vi "STA - Wave V6 Host_Wait.vi"() -> ()   [LabVIEW 2015]
doc: "The continuous acquisition mode tells the FPGA to acquire points indefinitely until a stop command is issued or until an error is encountered (FIFO overflow, module underflow, and so on). \n\nIn this acquisition mode, explicitly call the appropriate rwfm_ConfigTiming VI and set the host application's data buffer to be many times larger than the read size. The examples use a 10X size by default. If the host application's data buffer fills, then the FPGA experiences a FIFO overflow causing the acquisition to stop."
uses:
  <vilib>/rvi/interface/nirviCloseFPGA/nirviCloseFPGA.xnode
  <vilib>/FPGAPlugInAG/Dynamic/niLvFpga_Close_Dynamic.vi
  <vilib>/NI/cRIO Wfm/cRIO Wfm.lvlib
  <vilib>/rvi/interface/nirviMethod/nirviMethod.xnode
  <vilib>/rvi/interface/nirviMethod/StockFPGA_InlinedMethodWaitForSingleIRQ.vi
  <vilib>/FPGAPlugInAG/Dynamic/niLvFpga_WaitOnIrq_Dynamic.vi
  <vilib>/rvi/interface/nirviOpenFPGA/nirviOpenFPGA.xnode
  C:/Program Files (x86)/National Instruments/LabVIEW 2015/ProjectTemplates/Source/cRIOWfm/FPGA/[FPGA] SAR Acq Main.vi
  D/Documents/LabVIEW Data/STA - Waveform V0/FPGA Bitfiles/SARAcqMain_9074.lvbitx
  FPGA Bitfiles/STA-WaveformV6_FPGATarget2_[FPGA]DeltaSigMa_RDSJJgoi1gU.lvbitx
  FPGA/[FPGA] DeltaSig Main V6_bis.vi
  <vilib>/FPGAPlugInAG/cRIO-9112/niLvFpga_Open_cRIO-9112.vi
  <vilib>/rvi/interface/common/dynamic/niFpgaDynamicAddResources.vi
panel:
  out "Channel Config":T1(array[cluster])=[{"Channel Name"="Mod1/a0", "Sensitivity mV_EU"=1000.0, "EU"="V", "dB Ref EU"=1.0}, {"Channel Name"="Mod1/a1", "Sensitivity mV_EU"=1000.0, "EU"="V", "dB Ref EU"=1.0}, {"Channel Name"="Mod1/a2", "Sensitivity mV_EU"=1000.0, "EU"="V", "dB Ref EU"=1.0}, {"Channel Name"="Mod1/a3", "Sensitivity mV_EU"=1000.0, "EU"="V", "dB Ref EU"=1.0}, {"Channel Name"="Mod2/a0", "Sensitivity mV_EU"=1000.0, "EU"="V", "dB Ref EU"=1.0}, {"Channel Name"="Mod2/a1", "Sensitivity mV_EU"=1000.0, "EU"="V", "dB Ref EU"=1.0}, {"Channel Name"="Mod2/a2", "Sensitivity mV_EU"=1000.0, "EU"="V", "dB Ref EU"=1.0}, {"Channel Name"="Mod2/a3", "Sensitivity mV_EU"=1000.0, "EU"="V", "dB Ref EU"=1.0}, {"Channel Name"="Mod3/a0", "Sensitivity mV_EU"=1000.0, "EU"="V", "dB Ref EU"=1.0}, {"Channel Name"="Mod3/a1", "Sensitivity mV_EU"=1000.0, "EU"="V", "dB Ref EU"=1.0}, {"Channel Name"="Mod3/a2", "Sensitivity mV_EU"=1000.0, "EU"="V", "dB Ref EU"=1.0}, {"Channel Name"="Mod3/a3", "Sensitivity mV_EU"=1000.0, "EU"="V", "dB Ref EU"=1.0}, {"Channel Name"="Mod4/a0", "Sensitivity mV_EU"=1000.0, "EU"="V", "dB Ref EU"=1.0}, {"Channel Name"="Mod4/a1", "Sensitivity mV_EU"=1000.0, "EU"="V", "dB Ref EU"=1.0}, {"Channel Name"="Mod4/a2", "Sensitivity mV_EU"=1000.0, "EU"="V", "dB Ref EU"=1.0}, {"Channel Name"="Mod4/a3", "Sensitivity mV_EU"=1000.0, "EU"="V", "dB Ref EU"=1.0}, {"Channel Name"="Mod5/a0", "Sensitivity mV_EU"=1000.0, "EU"="V", "dB Ref EU"=1.0}, {"Channel Name"="Mod5/a1", "Sensitivity mV_EU"=1000.0, "EU"="V", "dB Ref EU"=1.0}, {"Channel Name"="Mod5/a2", "Sensitivity mV_EU"=1000.0, "EU"="V", "dB Ref EU"=1.0}, {"Channel Name"="Mod5/a3", "Sensitivity mV_EU"=1000.0, "EU"="V", "dB Ref EU"=1.0}, {"Channel Name"="Mod6/a0", "Sensitivity mV_EU"=1000.0, "EU"="V", "dB Ref EU"=1.0}, {"Channel Name"="Mod6/a1", "Sensitivity mV_EU"=1000.0, "EU"="V", "dB Ref EU"=1.0}, {"Channel Name"="Mod6/a2", "Sensitivity mV_EU"=1000.0, "EU"="V", "dB Ref EU"=1.0}, {"Channel Name"="Mod6/a3", "Sensitivity mV_EU"=1000.0, "EU"="V", "dB Ref EU"=1.0}] caption="Channel Name      Scale [mV/EU]              EU                           dB Ref [EU]"
  out "Time Measure":dbl
  out "data rate (S/s)":u32
  out "Samples per Read":i32
  out "file path":path
  out "error out":errorcluster
  in  "stop":bool
  out "Waveform Graph":waveform(sgl)[](graph)
  out "Buffer Backlog":dbl caption="RT Buffer Backlog [%]" format="%#.2g"
  # "Sampling Info"
  # "Channel Info"
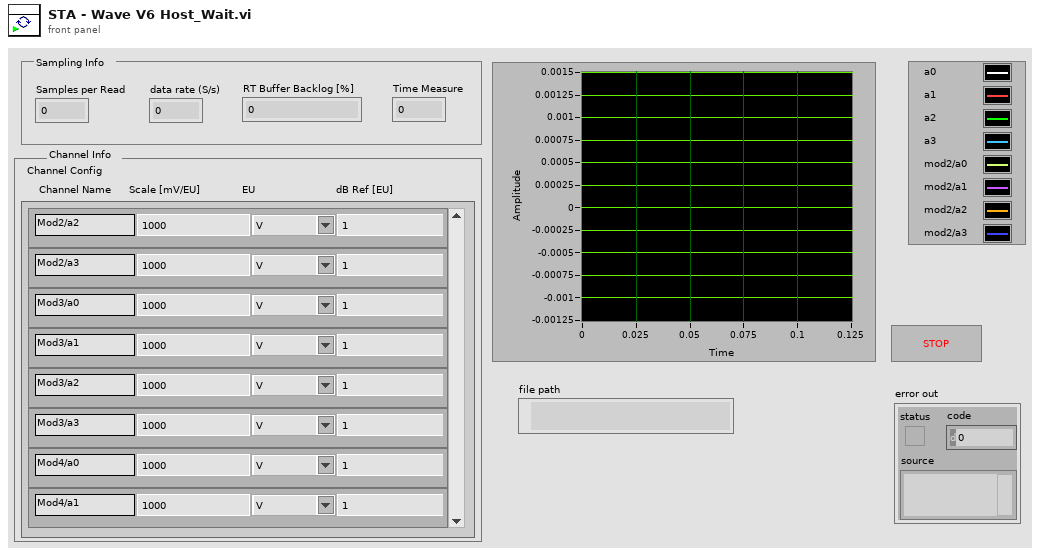
[diagram p1: front panel]
types:
  T1 = cluster{"Channel Name":string, "Sensitivity mV_EU":dbl, "EU":string, "dB Ref EU":dbl}[]
  T2 = enum16{"open", "open or create", "create or replace", "create", "open (read-only)"}
  T3 = typedef "nicrio_cRIO-9234_DataRatesRing2.ctl" = u8
  T4 = typedef "TDMS Properties.ctl" = cluster{"Name":string, "Value":string}
  T5 = typedef "nicrio_cRIO-9234_ConfigModeRing.ctl" = u8
  T6 = cluster{"Data Rate":T3, "Samples per Read":i32, "Number of Reads to Save":i32, "Data File Name":string, "TDMS Properties":T4[], "Number of Channels":i32, "Trigger - RMS Value":dbl, "Trigger - Channel":i32, "Trigger - Time (Minute)":i32, "data rate (S/s)":u32, "Time Measure":dbl, "Channel Config":cluster{"Channel Name":string, "Sensitivity mV_EU":dbl, "EU":string, "dB Ref EU":dbl}[], "Configuration Sensor":T5[]}
  T7 = typedef "cRIO Wfm.lvlib/SamplingInfo.ctl" = cluster{"Number of Channels":i32, "Actual Samp Rate":dbl, "Chan Name Array":string[], "EU Chan Array":string[], "dB Ref Chan Array":dbl[]}
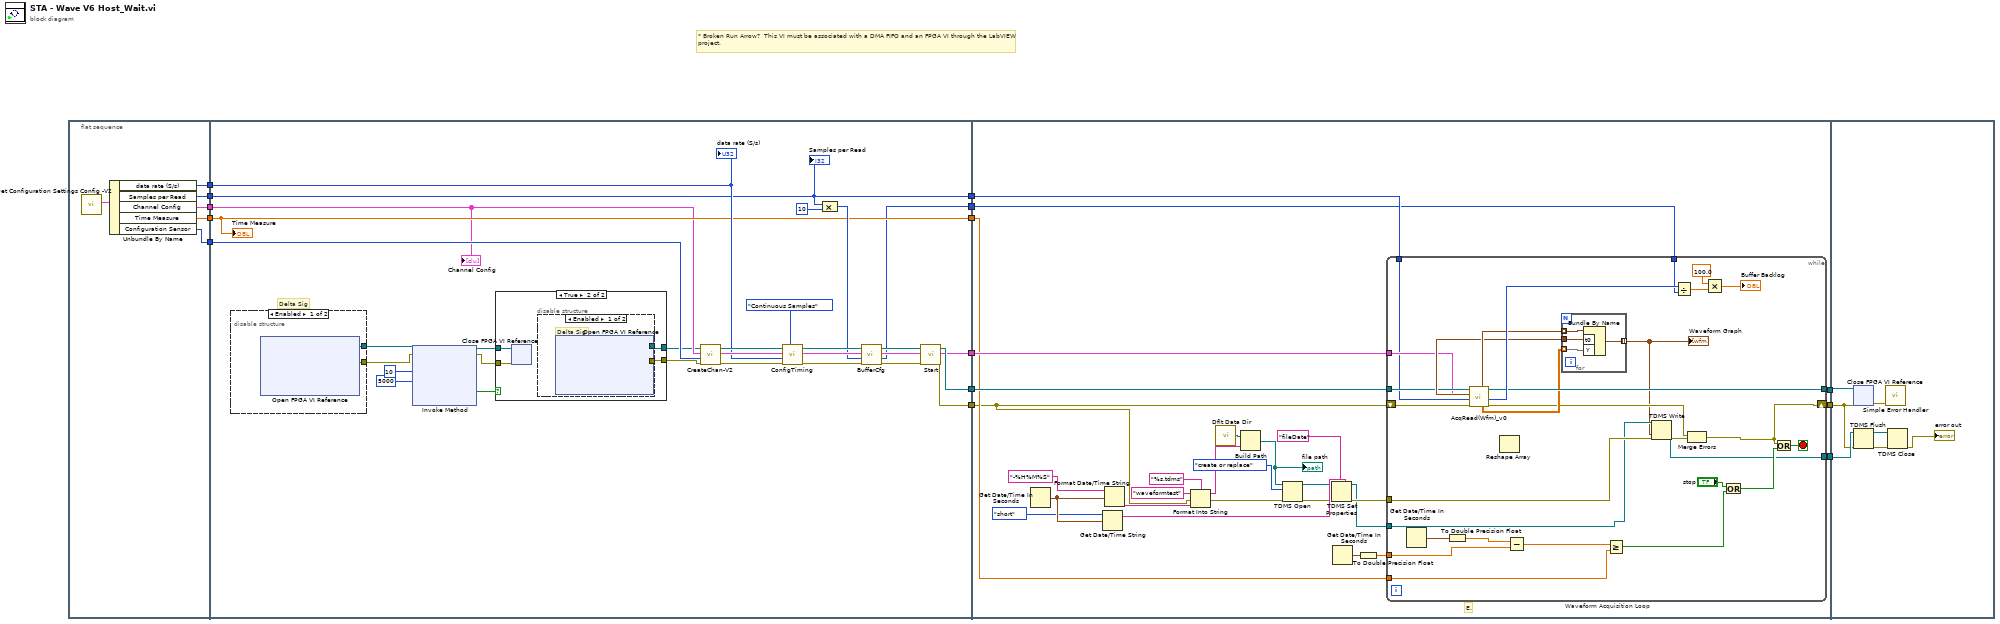
[diagram p0: block diagram]
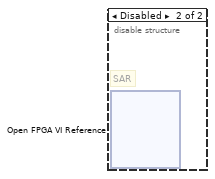
[diagram p2: hidden frame]
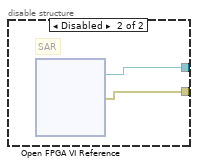
[diagram p4: hidden frame]
diagram:
  # "* Broken Run Arrow?  This VI must be associated with a DMA FIFO and an FPGA VI through the LabVIEW project."
  n1 = flat-sequence {
    tunnel: [w20] -> w14
    tunnel: [w19] -> w13
    tunnel: [w18] -> w12
    tunnel: [w17] -> w11
    tunnel: [w15] -> w1
    tunnel: w14 -> [w32]
    tunnel: w13 -> [w26]
    tunnel: w12 -> [w22]
    tunnel: w11 -> [w25]
    tunnel: [w26] -> w10
    tunnel: [w25] -> w9
    tunnel: [w29] -> w8
    tunnel: [w28] -> w7
    tunnel: [w27] -> w6
    tunnel: [w24] -> w5
    tunnel: w1 -> [w23]
    tunnel: w10 -> [w67]
    tunnel: w9 -> [w69]
    tunnel: w8 -> [w71]
    tunnel: w7 -> [w70]
    tunnel: w6 -> [w65]
    tunnel: w5 -> [w66]
    tunnel: [w74] -> w4
    tunnel: [w73] -> w3
    tunnel: [w72] -> w2
    tunnel: w4 -> [w128]
    tunnel: w3 -> [w126]
    tunnel: w2 -> [w127]
    frame #0 {
      n2 = call "Get Configuration Settings Config -V2.vi"() -> ("Acquisition and Logging Configuration"=w16:T6)  [unwired: 10 in, 1 out]
      n3 = Unbundle By Name(w16) -> ("data rate (S/s)"=w20:u32, "Samples per Read"=w19:i32, "Channel Config"=w18:T1, "Time Measure"=w17:dbl, "Configuration Sensor"=w15:T5[])
    }
    frame #1 {
      # "Delta Sig"
      n4 = disable-structure shown="Enabled" {
        disable-tunnel: [w52 _] -> w31
        disable-tunnel: [w51 _] -> w30
        frame Enabled {
          n5 = xnode "Open FPGA VI Reference"() -> ("FPGA VI Reference Out"=w52:refnum<k20>, "error out"=w51:errorcluster)  [unwired: 2 in]
        }
        frame Disabled {
          # "SAR"
          n6 = xnode "Open FPGA VI Reference"() -> ("FPGA VI Reference Out"=w54:refnum<k20>, "error out"=w53:errorcluster)  [unwired: 2 in]
        }
      }
      n7 = xnode "Invoke Method"("FPGA VI Reference In"=w31, "error in"=w30, "IRQ Number(s)"=10, "Timeout (ms)"=5000) -> ("FPGA VI Reference Out"=w48:refnum<k20>, "error out"=w49:errorcluster, "Timed Out"=w47:bool)  [unwired: 1 out]
      n8 = case shown="True" w47 {
        tunnel: w48 -> [w56 w60]
        tunnel: w49 -> [w55 w59]
        tunnel: [w56 w58] -> w21
        tunnel: [w55 w57] -> w50
        frame False {
        }
        frame True {
          n9 = xnode "Close FPGA VI Reference"("FPGA VI Reference In"=w60, "error in"=w59) -> ()  [unwired: 1 out]
          n10 = disable-structure shown="Enabled" {
            disable-tunnel: [w62 w64] -> w58
            disable-tunnel: [w61 w63] -> w57
            frame Enabled {
              # "Delta Sig"
              n11 = xnode "Open FPGA VI Reference"() -> ("FPGA VI Reference Out"=w62:refnum<k20>, "error out"=w61:errorcluster)  [unwired: 2 in]
            }
            frame Disabled {
              # "SAR"
              n12 = xnode "Open FPGA VI Reference"() -> ("FPGA VI Reference Out"=w64:refnum<k20>, "error out"=w63:errorcluster)  [unwired: 2 in]
            }
          }
        }
      }
      n13 = call "CreateChan-V2.vi"("Dynamic FPGA Ref"=w21, "Channel Config"=w22, "Configuration Sensor"=w23, "error in"=w50) -> ("Dynamic FPGA Ref Out"=w38:refnum<k20>, "Sampling Info"=w39:T7, "error out"=w43:errorcluster)  [unwired: 4 in]
      n14 = call <vilib>:"ConfigTiming.vi"("Sample Mode"=enum16{"Finite Samples", "Continuous Samples"}."Continuous Samples", "error in"=w43, "Sample Rate"=w32, "Sampling Info In"=w39, "Dynamic FPGA Ref"=w38) -> ("error out"=w42:errorcluster, "Sampling Info Out"=w41:T7, "Dynamic FPGA Ref Out"=w40:refnum<k20>)  [unwired: 3 in, 1 out]
      n15 = Compound Arithmetic op=MULTIPLY(w26, 10 ("value")) -> (w36:i32)
      n16 = call <vilib>:"BufferCfg.vi"("error in"=w42, "Buffer Size [Samps per Chan]"=w36, "Sampling Info In"=w41, "Dynamic FPGA Ref"=w40) -> ("error out"=w35:errorcluster, "Buffer Size [Total Samples]"=w24:u32, "Sampling Info Out"=w37:T7, "Dynamic FPGA Ref Out"=w34:refnum<k20>)  [unwired: 4 out]
      n17 = call <vilib>:"Start.vi"("error in"=w35, "Sampling Info In"=w37, "Dynamic FPGA Ref"=w34) -> ("error out"=w27:errorcluster, "Sampling Info Out"=w28:T7, "Dynamic FPGA Ref Out"=w29:refnum<k20>)  [unwired: 6 out]
      "Samples per Read" <- w26
      "data rate (S/s)" <- w32
      "Time Measure" <- w25
      "Channel Config" <- w22
    }
    frame #2 {
      # "E."
      n18 = Get Date/Time In Seconds() -> (seconds since 1Jan1904=w89:timestamp)
      n19 = Get Date/Time String(date format (0)=enum16{"short", "long", "abbreviated"}."short", seconds (now)=w89) -> (date string=w92:string)  [unwired: 1 in, 1 out]
      n20 = Format Date/Time String(time format string (%c)="-%H%M%S", seconds (now)=w89) -> (date/time string=w79:string)  [unwired: 1 in]
      n21 = Format Into String(format string="%s.tdms", initial string="waveformtest", error in=w65, w79) -> (resulting string=w75:string, error out=w86:errorcluster)
      n22 = call <vilib>:"Dflt Data Dir.vi"() -> ("App:Default Data Directory"=w80:path)
      n23 = Build Path(base path=w80, name or relative path=w75) -> (appended path=w83:path)
      "file path" <- w83
      n24 = TDMS Open(8:w86, 10:T2."create or replace" ("operation (0:open)"), 11:w83) -> (0:w81:errorcluster, 3:w82:refnum<k34>)  [unwired: 4 in]
      n25 = TDMS Set Properties(5:w92, 7:"fileDate" ("property names"), 8:w81, 11:w82) -> (0:w88:errorcluster, 3:w87:refnum<k34>)  [unwired: 2 in, 2 out]
      n26 = Get Date/Time In Seconds() -> (seconds since 1Jan1904=w91:timestamp)
      n27 = To Double Precision Float(number=w91) -> (double precision float=w90:dbl)
      n28 = while "Waveform Acquisition Loop" {
        tunnel: [w115] -> w74
        shift-right: [w110] -> w73
        shift-left: w65 -> [w121]
        tunnel: w87 -> [w96]
        tunnel: w88 -> [w97]
        tunnel: [w95] -> w72
        tunnel: w90 -> [w103]
        tunnel: w69 -> [w102]
        tunnel: w71 -> [w101]
        tunnel: w70 -> [w100]
        tunnel: w67 -> [w99]
        tunnel: w66 -> [w98]
        stop <- w116 stop-if-true
        n29 = Get Date/Time In Seconds() -> (seconds since 1Jan1904=w105:timestamp)
        n30 = To Double Precision Float(number=w105) -> (double precision float=w104:dbl)
        n31 = call <vilib>:"AcqRead(Wfm)_v0.vi"("error in"=w121, "Samps Read per Chan"=w99, "Sampling Info"=w100, "Dynamic FPGA Ref"=w101) -> ("error out"=w111:errorcluster, "Samples Remaining"=w120:u32, "time stamp"=w112:timestamp, "Dynamic FPGA Ref Out"=w115:refnum<k20>, "transposed array"=w113:sgl[][], "Array"=w114:waveform(sgl)[])  [unwired: 2 in]
        n32 = Reshape Array() -> ()  [unwired: 2 in, 1 out]
        n33 = Subtract(x=w104, y=w103) -> (x-y=w106:dbl)
        n34 = for {
          tunnel: w114 -> [w125] mode=indexing
          tunnel: w112 -> [w124]
          tunnel: [w123] -> w94 mode=indexing
          tunnel: w113 -> [w122] mode=indexing
          n35 = Bundle By Name(cluster=w125, "t0"=w124, "Y"=w122) -> (w123:waveform(sgl))
        }
        "Waveform Graph" <- w94
        n36 = Greater Or Equal?(x=w106, y=w102) -> (x >= y?=w109:bool)
        n37 = TDMS Write(0:w96, 9:w94, 11:w97) -> (4:w95:refnum<k34>, 15:w93:errorcluster)  [unwired: 3 in, 2 out]
        n38 = Divide(x=w120, y=w98) -> (x/y=w119:dbl)
        n39 = Merge Errors(w111, w93) -> (w110:errorcluster)
        n40 = Multiply(x=100.0, y=w119) -> (x*y=→"Buffer Backlog":dbl)
        n41 = Or(x="stop", y=w109) -> (x .or. y?=w107:bool)
        n42 = Or(x=w110, y=w107) -> (x .or. y?=w116:bool)
      }
    }
    frame #3 {
      n43 = xnode "Close FPGA VI Reference"("FPGA VI Reference In"=w128, "error in"=w126) -> ("error out"=w129:errorcluster)
      n44 = TDMS Flush(4:w126, 7:w127) -> (0:w130:errorcluster, 3:w132:refnum<k34>)
      n45 = call <vilib>:"Simple Error Handler.vi"("error in (no error)"=w129) -> ()  [unwired: 1 in, 8 out]
      n46 = TDMS Close(8:w130, 11:w132) -> (0:→"error out":errorcluster)  [unwired: 1 out]
    }
  }
